vi "Teleop - Trigger (SubVI).vi"(1 "Trigger":bool) -> (0 "Trigger Output":bool)   [LabVIEW 2020]
doc: "The trigger VI is design to send a true output for only 1 loop after the input has gone true. To reset the trigger, the input must go false before it goes true again."
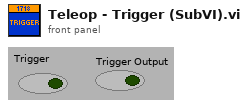
[diagram p1: front panel]
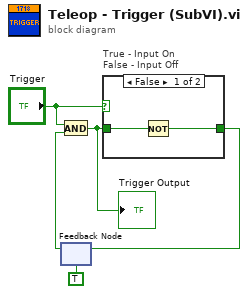
[diagram p0: block diagram]
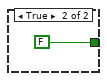
[diagram p2: hidden frame]
diagram:
  n1 = feedback #1(TRUE) -> (w3:bool)
  n2 = And(x="Trigger", y=w3) -> (x .and. y?=w4:bool)
  "Trigger Output" <- w4
  n3 = case "True - Input On\nFalse - Input Off" shown="False" "Trigger" {
    tunnel: w4 -> [w7 _]
    tunnel: [w6 FALSE] -> w5
    frame False {
      n4 = Not(x=w7) -> (.not. x?=w6:bool)
    }
    frame True {
    }
  }
  n5 = feedback-in #1(w5) -> ()
